vi "Cosine Tapered Window (CDB).vi"(10 "ratio":dbl=0.2, 11 "X":cdb[](array[numeric])) -> (0 "error":i32, 3 "Windowed X":cdb[](array[numeric]))   [LabVIEW 2017, in "NI_AALPro.lvlib"]
doc: "Applies a cosine tapered window to the input sequence <B>X</B>. Wire data to the <B>X</B> input to determine the polymorphic instance to use or manually select the instance."
uses:
  NI_AALPro.lvlib
  lvanlys.dll
panel:
  # "Cosine Tapered Window"
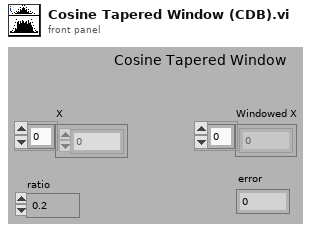
[diagram p1: front panel]
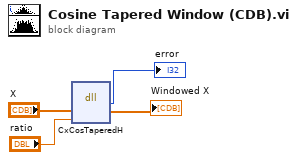
[diagram p0: block diagram]
diagram:
  n1 = dll-call lib="C:/Program Files/National Instruments/LabVIEW 2017/resource/lvanlys.*" fn="CxCosTaperedH"("X"="X", "r"="ratio") -> (→"error":i32, "X"=→"Windowed X":cdb[])  [unwired: 4 in, 2 out]
